vi "get CloudComputerName.vi"(8 "error in (no error)":errorcluster caption="错误输入（无错误）") -> (0 "error out":errorcluster caption="错误输出", 3 "String/Binary data":string caption="CloudComputerName")   [LabVIEW 2022 SP3]
uses:
  <vilib>/registry/registry.llb/Registry RtKey.ctl
  <vilib>/registry/registry.llb/Registry SAM.ctl
  <vilib>/registry/registry.llb/Read Registry Value Simple STR.vi
panel:
  out "subkey":string
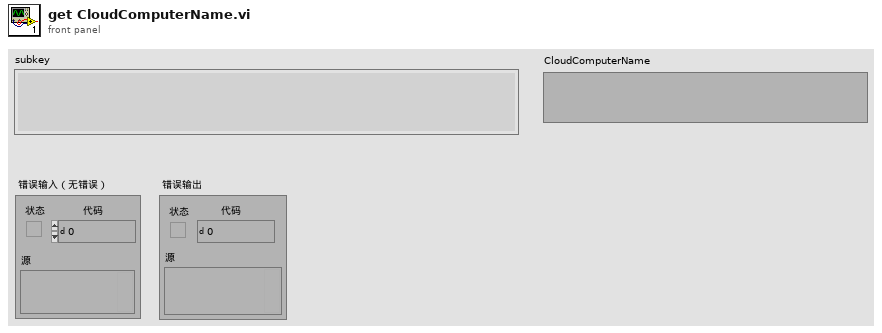
[diagram p1: front panel]
types:
  T1 = typedef "Registry SAM.ctl" = enum32{"KEY_QUERY_VALUE", "KEY_SET_VALUE", "KEY_CREATE_SUB_KEY", "KEY_ENUMERATE_SUB_KEYS", "KEY_NOTIFY", "KEY_CREATE_LINK", "KEY_READ", "KEY_WRITE", "KEY_ALL_ACCESS", "KEY_READ | KEY_WRITE"}
  T2 = typedef "Registry RtKey.ctl" = enum32{"HKEY_CLASSES_ROOT", "HKEY_CURRENT_USER", "HKEY_LOCAL_MACHINE", "HKEY_USERS", "HKEY_PERFORMANCE_DATA", "HKEY_CURRENT_CONFIG", "HKEY_DYN_DATA"}
  T3 = typedef "Registry refnum.ctl" = refnum<k1>
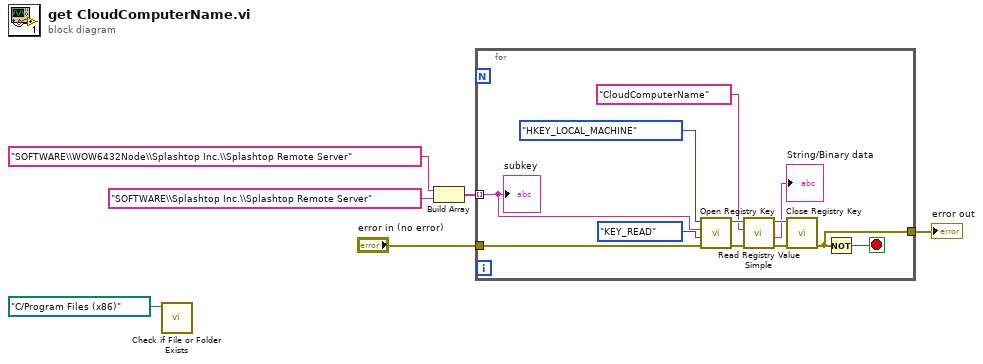
[diagram p0: block diagram]
diagram:
  n1 = call <vilib>:"Check if File or Folder Exists.vi"("path"=path "C:/Program Files (x86)") -> ()  [unwired: 8 in, 3 out]
  n2 = Build Array("SOFTWARE\\WOW6432Node\\Splashtop Inc.\\Splashtop Remote Server" ("subkey"), "SOFTWARE\\Splashtop Inc.\\Splashtop Remote Server" ("subkey")) -> (w3:string[])
  n3 = for {
    tunnel: w3 -> [w9] mode=indexing
    tunnel: "error in (no error)" -> [w15]
    tunnel: [w7] -> w5
    stop <- w8 stop-if-true
    n4 = call <vilib>:"Open Registry Key.vi"("error in (no error)"=w15, "security access mask (KEY_READ | KEY_WRITE)"=Registry_SAM."KEY_READ", "subkey"=w9, "root key (HKEY_LOCAL_MACHINE)"=Registry_RtKey."HKEY_LOCAL_MACHINE") -> ("error out"=w12:errorcluster, "refnum out"=w13:T3)  [unwired: 6 in]
    n5 = call-poly <vilib>:"Read Registry Value Simple.vi"("error in (no error)"=w12, "value"="CloudComputerName", "refnum"=w13) -> ("error out"=w16:errorcluster, "String/Binary data"=→"String/Binary data":string, "refnum out"=w17:T3)  [unwired: 3 in, 1 out]
    n6 = call <vilib>:"Close Registry Key.vi"("error in (no error)"=w16, "refnum"=w17) -> ("error out"=w7:errorcluster)  [unwired: 5 in]
    n7 = Not(x=w7) -> (.not. x?=w8:bool)
    "subkey" <- w9
  }
  "error out" <- w5
